vi "Modbus Life Bit Toggle.vi"(10 "Toggle Input":bool, 11 "seconds since 1Jan1904 in":timestamp) -> (2 "Toggle Output":bool, 3 "seconds since 1Jan1904 out":timestamp)   [LabVIEW 2020, in "Modbus.lvlib"]
uses:
  Modbus.lvlib
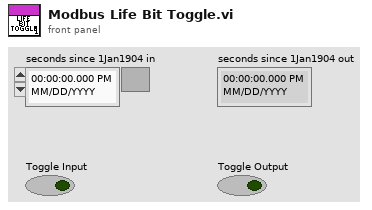
[diagram p1: front panel]
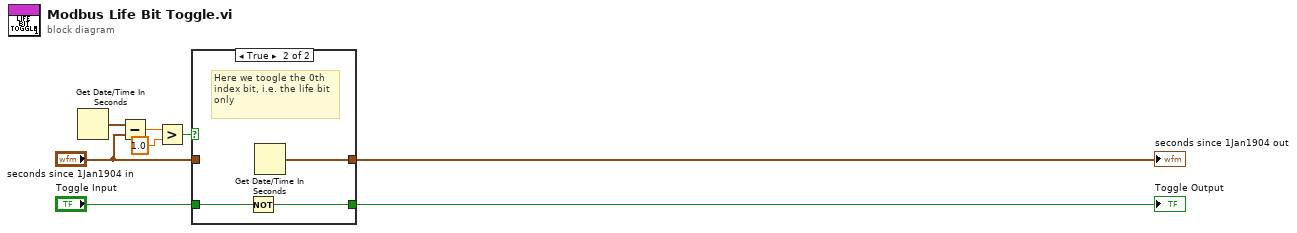
[diagram p0: block diagram]
diagram:
  n1 = Get Date/Time In Seconds() -> (seconds since 1Jan1904=w1:timestamp)
  n2 = Subtract(x=w1, y="seconds since 1Jan1904 in") -> (x-y=w2:dbl)
  n3 = Greater?(x=w2, y=1.0) -> (0:w4:bool)
  n4 = case shown="True" w4 {
    tunnel: "seconds since 1Jan1904 in" -> [w9 _]
    tunnel: [w9 w13] -> w5
    tunnel: "Toggle Input" -> [w10 w12]
    tunnel: [w10 w11] -> w8
    frame False {
    }
    frame True {
      # "Here we toogle the 0th index bit, i.e. the life bit only"
      n5 = Not(x=w12) -> (.not. x?=w11:bool)
      n6 = Get Date/Time In Seconds() -> (seconds since 1Jan1904=w13:timestamp)
    }
  }
  "Toggle Output" <- w8
  "seconds since 1Jan1904 out" <- w5
